vi "Test Process Multiple Start.vi"(8 "error in (no error)":errorcluster, 11 "Process Test In":refnum<class "Process Test.lvclass">) -> (0 "error out":errorcluster, 3 "Process Test Out":refnum<class "Process Test.lvclass">)   [LabVIEW 2020, in "Process Test.lvclass"]
uses:
  Process Test.lvclass
  C:/Program Files (x86)/National Instruments/LabVIEW 2020/vi.lib/Asteme/LUnit/Test Case.lvclass
  Mock Error Handler/Mock Error Handler.lvclass
  C:/Users/anton/Documents/GitHub/Triarc-Framework/source/Framework/Process/Process.lvclass
  C:/Users/anton/Documents/GitHub/Triarc-Framework/source/Framework/Error Handler Interface/Error Handler Interface.lvclass
  Framework/Process/Process.lvclass/Process.ctl
  <vilib>/Asteme/LUnit/Test Case.lvclass/Test Case.ctl
  <vilib>/Asteme/LUnit/LUnit Assertion Result.lvclass/LUnit Assertion Result.ctl
  Framework/Process/Public/Lifecycle/Get Lifecycle State.vi
  Framework/Process/Protected/Messaging/Enqueue Message.vi
  <vilib>/Utility/error.llb/Clear Errors.vi
  <vilib>/Asteme/LUnit/Palette/Pass.vi
  <vilib>/Asteme/LUnit/Palette/Fail.vi
  <vilib>/Asteme/LUnit/Set Assertion Type.vi
  Framework/Process/Private/SubVIs/Wait for finish.vi
  Framework/Process/Private/SubVIs/Set Lifecycle State.vi
  <vilib>/AdvancedString/1D String Array to Delimited String.vi
  <vilib>/Asteme/LUnit/Add test result.vi
  <vilib>/Asteme/LUnit/LUnit Write Passed.vi
  <vilib>/Asteme/LUnit/LUnit Get Test Case.vi
  <vilib>/Asteme/LUnit/LUnit Write Message.vi
  <vilib>/Asteme/LUnit/LUnit Write Description.vi
  <vilib>/Asteme/LUnit/LUnit Write Assertion Type.vi
  <vilib>/Asteme/LUnit/Read Test Case Name.vi
  <vilib>/Utility/error.llb/Error Cluster From Error Code.vi
  <vilib>/Asteme/LUnit/Assertion Result/LUnit Get Test Name.vi
  Framework/Process/Process.lvclass
  <vilib>/Asteme/LUnit/LUnit Assertion Result.lvclass
  <vilib>/Asteme/LUnit/Test Case.lvclass
  C:/Users/anton/Documents/GitHub/Triarc-Framework/source/Framework Test/Base Class Test/Base Test.lvclass
  C:/Users/anton/Documents/GitHub/Triarc-Framework/source/Framework Test/Process Test/Process Test.lvclass
  C:/Users/anton/Documents/GitHub/Triarc-Framework/source/Framework/Base/Base.lvclass
  C:/Users/anton/Documents/GitHub/Triarc-Framework/source/Framework Test/Mock Error Handler/Mock Error Handler.lvclass
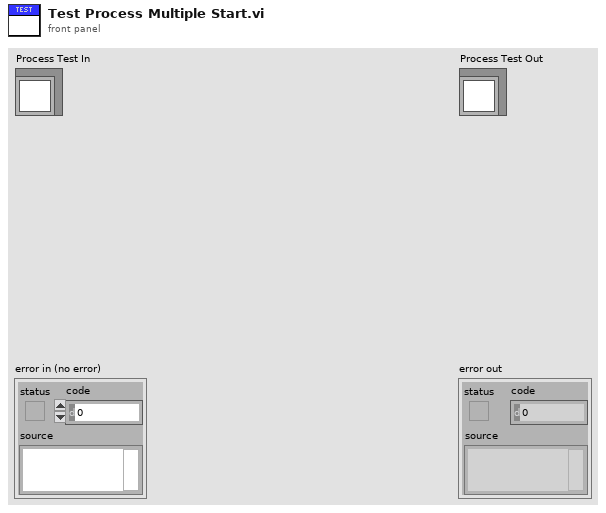
[diagram p1: front panel]
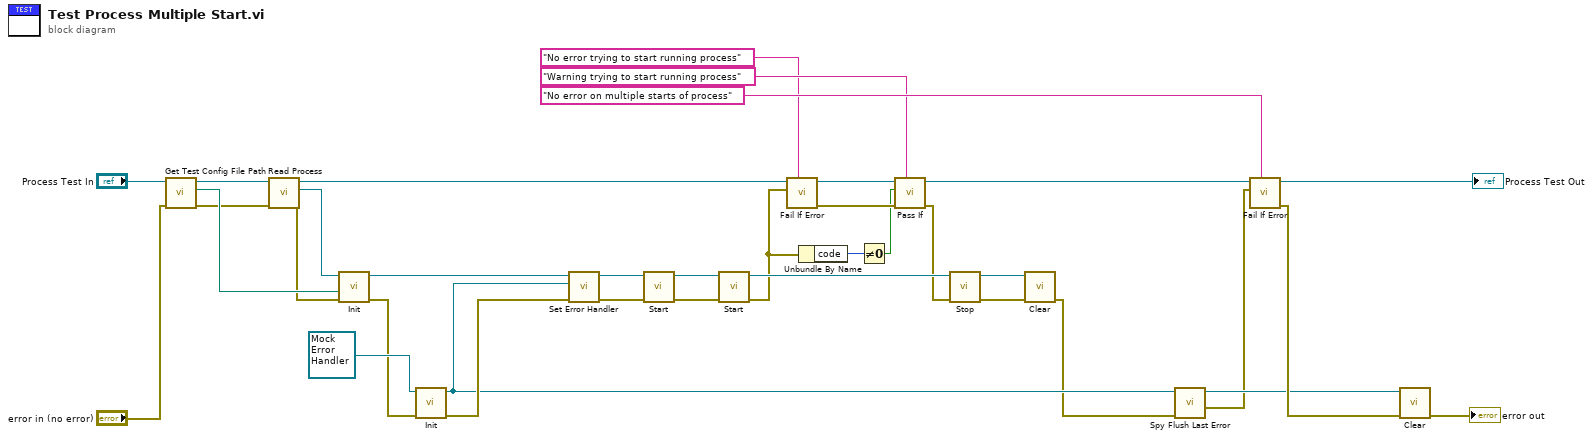
[diagram p0: block diagram]
diagram:
  n1 = call-dynamic "Get Test Config File Path.vi"("error in (no error)"="error in (no error)", "Base Class Test in"="Process Test In") -> ("error out"=w27:errorcluster, "Test config path"=w30:path, "Base Class Test out"=w32:refnum<class "Process Test.lvclass">)  [unwired: 7 in]
  n2 = call "Read Process.vi"("error in (no error)"=w27, "Process Test in"=w32) -> ("error out"=w28:errorcluster, "Process.lvclass"=w29:refnum<class "Process.lvclass">, "Process Test out"=w5:refnum<class "Process Test.lvclass">)  [unwired: 7 in]
  n3 = call-dynamic "Init.vi"("error in (no error)"=w28, "Config File Path"=w30, "Process In"=w29) -> ("error out"=w17:errorcluster, "Process Out"=w33:refnum<class "Process.lvclass">)  [unwired: 7 in]
  n4 = call-dynamic "Init.vi"("error in (no error)"=w17, "Mock Error Handler In"=refnum<class "Mock Error Handler.lvclass"> refnum ("Mock Error Handler.lvclass")) -> ("error out"=w21:errorcluster, "Mock Error Handler Out"=w20:refnum<class "Mock Error Handler.lvclass">)  [unwired: 8 in]
  n5 = call "Set Error Handler.vi"("error in (no error)"=w21, "Error Handler"=w20, "Process In"=w33) -> ("error out"=w22:errorcluster, "Process Out"=w23:refnum<class "Process.lvclass">)  [unwired: 7 in]
  n6 = call "Start.vi"("error in (no error)"=w22, "Process In"=w23) -> ("error out"=w35:errorcluster, "Process Out"=w36:refnum<class "Process.lvclass">)  [unwired: 8 in]
  n7 = call "Start.vi"("error in (no error)"=w35, "Process In"=w36) -> ("error out"=w4:errorcluster, "Process Out"=w26:refnum<class "Process.lvclass">)  [unwired: 8 in]
  n8 = call <vilib>:"Fail If Error.vi"("Description"="No error trying to start running process", "Assert error"=w4, "Test Case In"=w5) -> ("error out"=w10:errorcluster, "Test Case Out"=w11:refnum<class "Process Test.lvclass">)  [unwired: 7 in]
  n9 = Unbundle By Name(w4) -> ("code"=w9:i32)
  n10 = Not Equal To 0?(x=w9) -> (x != 0?=w8:bool)
  n11 = call <vilib>:"Pass If.vi"("Description"="Warning trying to start running process", "error in (no error)"=w10, "Pass?"=w8, "Test Case In"=w11) -> ("error out"=w3:errorcluster, "Test Case Out"=w2:refnum<class "Process Test.lvclass">)  [unwired: 6 in]
  n12 = call "Stop.vi"("error in (no error)"=w3, "Process In"=w26) -> ("error out"=w24:errorcluster, "Process Out"=w25:refnum<class "Process.lvclass">)  [unwired: 7 in, 1 out]
  n13 = call-dynamic "Clear.vi"("error in (no error)"=w24, "Process In"=w25) -> ("error out"=w16:errorcluster)  [unwired: 8 in, 1 out]
  n14 = call "Spy Flush Last Error.vi"("error in (no error)"=w16, "Mock Error Handler In"=w20) -> ("Error"=w1:errorcluster, "Mock Error Handler Out"=w14:refnum<class "Mock Error Handler.lvclass">)  [unwired: 7 in, 1 out]
  n15 = call <vilib>:"Fail If Error.vi"("Description"="No error on multiple starts of process", "Assert error"=w1, "Test Case In"=w2) -> ("error out"=w15:errorcluster, "Test Case Out"=→"Process Test Out":refnum<class "Process Test.lvclass">)  [unwired: 7 in]
  n16 = call-dynamic "Clear.vi"("error in (no error)"=w15, "Mock Process In"=w14) -> ("error out"=→"error out":errorcluster)  [unwired: 8 in, 1 out]
